vi "Main.vi"() -> ()   [LabVIEW 2017]
doc: "\"Discrete LED demo.vi\" -- Demonstrate a discrete LED connected to a digital output.\n\nInstructions:\n\n-- Click the 'enable blinker' button to toggle between blinking mode\nand static mode.\n-- In static mode, click the 'digital level' button to set the state of the\ndigital output.\n-- The 'digital output state' LED indicator shows the state of the\ndigital output (on = high, off = low)."
uses:
  <vilib>/myRIO/Instrument Drivers/Onboard IO/PWM/typedefs/PWM Reference.ctl
  <vilib>/myRIO/Common/Instrument Driver Framework/Utilities/typedefs/myRIO Generic Hardware Reference.ctl
  <vilib>/myRIO/Common/Instrument Driver Framework/Utilities/typedefs/Hardware Version Enum.ctl
  <vilib>/myRIO/Common/Instrument Driver Framework/Utilities/typedefs/myRIO v1.0 Reference.ctl
  <vilib>/myRIO/Common/Instrument Driver Framework/Utilities/typedefs/Generic FPGA Reference.ctl
  <vilib>/myRIO/Common/Instrument Driver Framework/myRIO v1.0/PWM/typedefs/PWM Channels Enum.ctl
  <vilib>/myRIO/Instrument Drivers/Onboard IO/PWM/typedefs/PWM Configuration.ctl
  <vilib>/userdefined/High Color/nirio_resource_hc.ctl
  <vilib>/myRIO/Instrument Drivers/Onboard IO/DIO/typedefs/DIO Reference.ctl
  <vilib>/myRIO/Common/Instrument Driver Framework/myRIO v1.0/DIO/typedefs/DIO Channels List.ctl
  <vilib>/myRIO/Common/Instrument Driver Framework/myRIO v1.0/DIO/typedefs/DIO Channels Enum.ctl
  <vilib>/myRIO/Common/Instrument Driver Framework/Utilities/vis/Is FPGA Ref Available.vi
  <vilib>/myRIO/Common/Instrument Driver Framework/myRIO v1.0/PWM/vis/myRIO v1.1 Open PWM.vi
  <vilib>/myRIO/Instrument Drivers/Onboard IO/PWM/vis/Set Duty Cycle and Frequency.vi
  <vilib>/myRIO/Common/Instrument Driver Framework/myRIO v1.0/DIO/vis/myRIO v1.1 Open DIO.vi
  <vilib>/myRIO/Instrument Drivers/Onboard IO/DIO/vis/Write.vi
  <vilib>/myRIO/Common/Instrument Driver Framework/Utilities/vis/Validate Channels.vi
  <vilib>/myRIO/Common/Instrument Driver Framework/myRIO v1.0/PWM/vis/myRIO v1.0 Reserve PWM.vi
  <vilib>/myRIO/Common/Instrument Driver Framework/myRIO v1.0/DIO/vis/myRIO v1.0 Reserve DIO.vi
  <vilib>/myRIO/Common/Instrument Driver Framework/myRIO v1.0/UART/vis/myRIO v1.0 Close UART.vi
  <vilib>/myRIO/Common/Instrument Driver Framework/myRIO v1.0/PWM/vis/myRIO v1.0 Build MUX Configuration PWM.vi
  <vilib>/myRIO/Common/Instrument Driver Framework/myRIO v1.0/Resource Manager/vis/myRIO v1.0 Reserve Channel List.vi
  <vilib>/myRIO/Common/Instrument Driver Framework/myRIO v1.0/DIO/vis/myRIO v1.0 Build MUX Configuration DIO.vi
  <vilib>/myRIO/Common/Instrument Driver Framework/myRIO v1.0/Resource Manager/vis/myRIO v1.0 Create Configuration List.vi
  <vilib>/myRIO/Common/Instrument Driver Framework/myRIO v1.0/Resource Manager/vis/myRIO v1.0 Reserve Channel.vi
  <vilib>/myRIO/Common/Instrument Driver Framework/myRIO v1.0/Resource Manager/vis/myRIO v1.0 Unreserve Channel.vi
  <vilib>/myRIO/Common/Instrument Driver Framework/myRIO v1.0/Resource Manager/vis/myRIO v1.0 Build Mutex Name.vi
  <vilib>/Utility/VariantDataType/GetNumericInfo.vi
  <vilib>/Utility/error.llb/Error Cluster From Error Code.vi
  <vilib>/myRIO/Common/Instrument Driver Framework/myRIO v1.0/myRIO v1.1 Open.vi
  <vilib>/myRIO/Common/Instrument Driver Framework/Utilities/vis/IO Manager.vi
  <vilib>/myRIO/Common/Instrument Driver Framework/Utilities/vis/Configuration Manager.vi
  <vilib>/myRIO/Common/Instrument Driver Framework/myRIO v1.0/Resource Manager/vis/myRIO v1.0 Configure IO.vi
  <vilib>/myRIO/Common/Instrument Driver Framework/myRIO v1.0/myRIO v1.0 Close.vi
  <vilib>/myRIO/Common/Instrument Driver Framework/myRIO v1.0/PWM/vis/myRIO v1.0 Write PWM.vi
  <vilib>/myRIO/Common/Instrument Driver Framework/myRIO v1.0/DIO/vis/myRIO v1.0 Write DIO.vi
  <vilib>/myRIO/Common/Instrument Driver Framework/Utilities/vis/FPGA Ref Manager.vi
  <vilib>/myRIO/Common/Instrument Driver Framework/myRIO v1.0/myRIO v1.0 Reset FPGA.vi
  <vilib>/myRIO/Common/Instrument Driver Framework/myRIO v1.0/IRQ/vis/myRIO v1.0 IRQ Info FGV.vi
  <vilib>/myRIO/Common/Instrument Driver Framework/myRIO v1.0/IRQ/vis/myRIO v1.0 Timer IRQ Info FGV.vi
  <vilib>/myRIO/Common/Instrument Driver Framework/myRIO v1.0/IRQ/vis/myRIO v1.0 ISR Agent.vi
  <vilib>/myRIO/Express VI/Onboard IO/PWM/PWM Express VI.xnode
  <vilib>/myRIO/Instrument Drivers/Onboard IO/PWM/vis/myRIO PWM Open.xnode
  <vilib>/myRIO/Express VI/Onboard Devices/LED/LED Express VI.xnode
  <vilib>/myRIO/Instrument Drivers/Onboard IO/DIO/vis/myRIO DIO Open.xnode
  <vilib>/myRIO/Express VI/Onboard IO/DO/DO Express VI.xnode
  <vilib>/myRIO/Instrument Drivers/Utilities/Utilities.lvlib
  <vilib>/myRIO/Instrument Drivers/Onboard IO/PWM/PWM.lvlib
  <vilib>/myRIO/Instrument Drivers/Onboard IO/DIO/DIO.lvlib
panel:
  in  "millisecond timer value":u32=100
  in  "PWM 2":dbl(slide)=0.5 scale=0.0..1.0
  in  "PWM 1":dbl(slide)=0.5 scale=0.0..1.0
  in  "Stop Button":bool
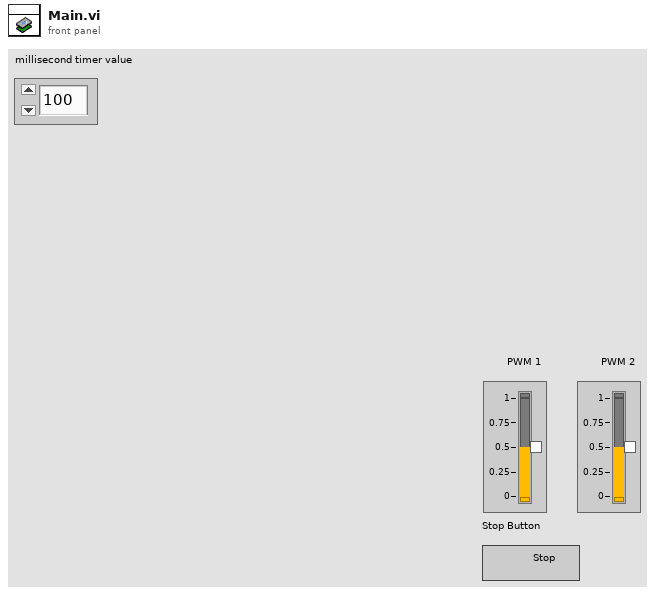
[diagram p1: front panel]
types:
  T1 = enum16{"0", "1", "2", "3", "4", "5", "6", "7", "8", "9", "A", "B", "C", "D", "E", "F", "G", "H", "I", "J", "K", "L", "M", "N", "O", "P", "Q", "R", "S", "T", "U", "V", "W", "X", "Y", "Z", "F1", "F2", "F3", "F4", "F5", "F6", "F7", "F8", "F9", "F10", "F11", "F12", "F13", "F14", "F15", "ADD", "BACK", "BACKSLASH", "CAPITAL", "COMMA", "DECIMAL", "DELETE", "DIVIDE", "DOWN", "END", "EQUALS", "ESCAPE", "GRAVE (`)", "HOME", "INSERT", "LBRACKET", "LCONTROL", "LEFT", "L ALT", "LSHIFT", "LWIN", "MINUS", "MULTIPLY", "NEXT", "NUMLOCK", "NUMPAD_0", "NUMPAD_1", "NUMPAD_2", "NUMPAD_3", "NUMPAD_4", "NUMPAD_5", "NUMPAD_6", "NUMPAD_7", "NUMPAD_8", "NUMPAD_9", "PAUSE", "PERIOD", "PRIOR (PG UP)", "RBRACKET", "RCONTROL", "RETURN", "RIGHT", "R ALT", "RSHIFT", "RWIN", "SCROLL", "SEMICOLON", "SLASH", "SPACE", "SUBTRACT", "TAB", "UP", "ENTER (num pad)", "' (quote)"}
  T2 = typedef "DIO.lvlib/DIO Reference.ctl" = cluster{"myRIO Reference":T3, "DIO Channels List":T7}
  T3 = typedef "myRIO Generic Hardware Reference.ctl" = cluster{"myRIO Model":T4, "myRIO Hardware Reference":T5}
  T4 = typedef "Hardware Version Enum.ctl" = enum16{"Unknown", "myRIO-1900", "myRIO-1950", "roboRIO", "NI ELVIS RIO CM"}
  T5 = typedef "myRIO v1.0 Reference.ctl" = cluster{"Generic FPGA Reference":T6, "Allow multiple opens":bool}
  T6 = typedef "Generic FPGA Reference.ctl" = refnum<k20>
  T7 = typedef "DIO Channels List.ctl" = T8[]
  T8 = typedef "DIO Channels Enum.ctl" = enum16{"Not Connected", "C/DIO0", "C/DIO1", "C/DIO2", "C/DIO3", "C/DIO4", "C/DIO5", "C/DIO6", "C/DIO7", "A/DIO0", "A/DIO1", "A/DIO2", "A/DIO3", "A/DIO4", "A/DIO5", "A/DIO6", "A/DIO7", "A/DIO8", "A/DIO9", "A/DIO10", "A/DIO11", "A/DIO12", "A/DIO13", "A/DIO14", "A/DIO15", "B/DIO0", "B/DIO1", "B/DIO2", "B/DIO3", "B/DIO4", "B/DIO5", "B/DIO6", "B/DIO7", "B/DIO8", "B/DIO9", "B/DIO10", "B/DIO11", "B/DIO12", "B/DIO13", "B/DIO14", "B/DIO15", "LED0", "LED1", "LED2", "LED3", "Button0", "DIO/DIO0", "DIO/DIO1", "DIO/DIO2", "DIO/DIO3", "DIO/DIO4", "DIO/DIO5", "DIO/DIO6", "DIO/DIO7", "DIO/DIO8", "DIO/DIO9", "SPI/CS0", "SPI/CS1", "SPI/CS2", "SPI/CS3", "LED RADIO (Green)", "LED RADIO (Red)", "LED COMM (Green)", "LED COMM (Red)", "LED MODE (Green)", "LED MODE (Red)"}
  T9 = typedef "nirio_resource_hc.ctl" = tag
  T10 = typedef "PWM.lvlib/PWM Reference.ctl" = cluster{"myRIO Reference":T3, "PWM Channels Enum":T11, "PWM Configuration":T12}
  T11 = typedef "PWM Channels Enum.ctl" = enum16{"Not Connected", "C/PWM0", "C/PWM1", "A/PWM0", "A/PWM1", "A/PWM2", "B/PWM0", "B/PWM1", "B/PWM2", "PWM/PWM0", "PWM/PWM1", "PWM/PWM2", "PWM/PWM3", "PWM/PWM4", "PWM/PWM5", "PWM/PWM6", "PWM/PWM7", "PWM/PWM8", "PWM/PWM9"}
  T12 = typedef "PWM.lvlib/PWM Configuration.ctl" = cluster{"Frequency":dbl, "Duty Cycle":dbl}
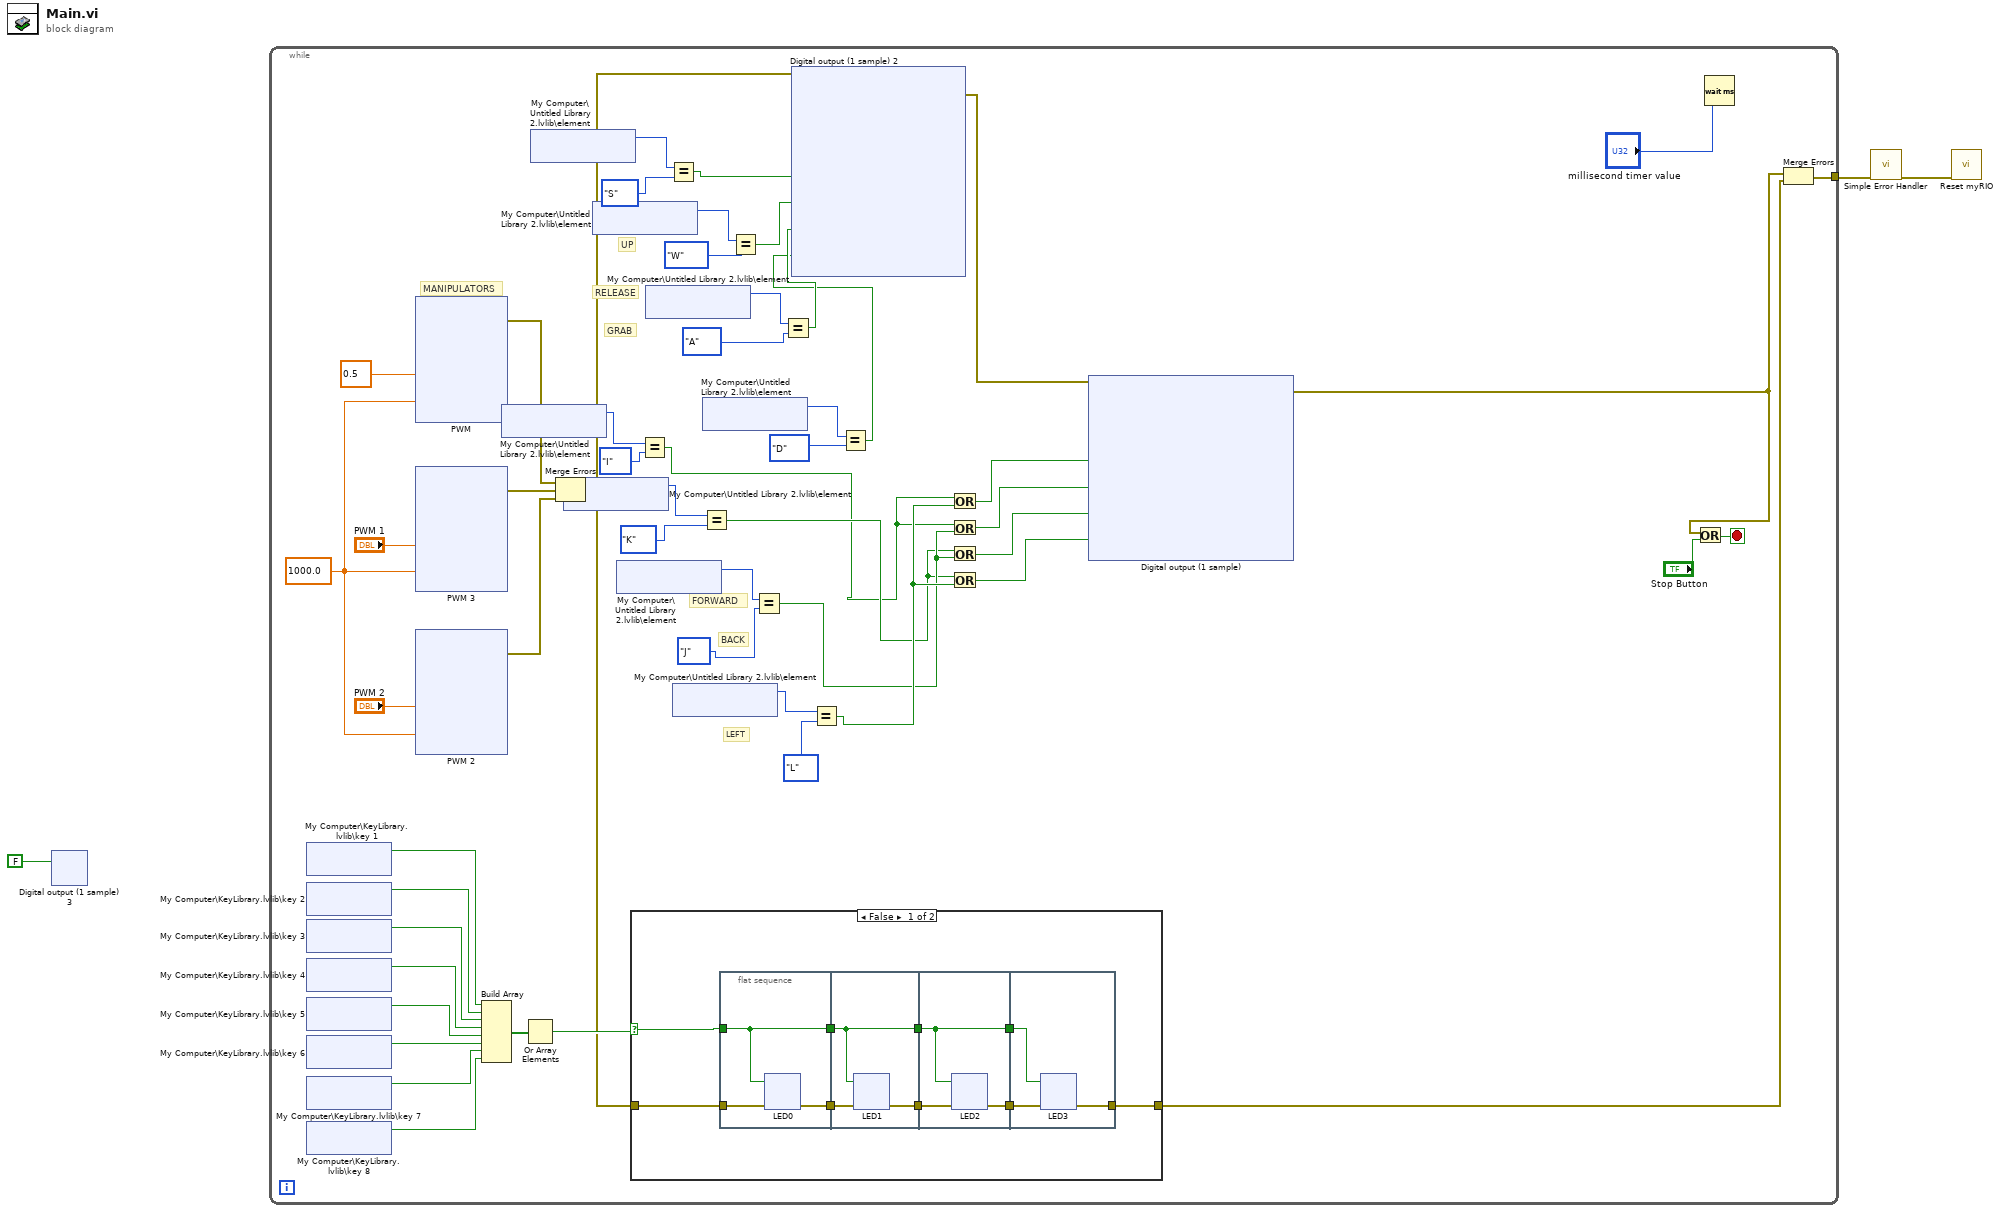
[diagram p0: block diagram]
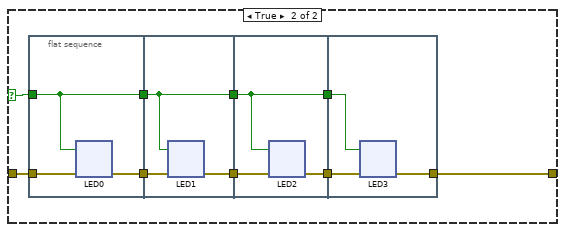
[diagram p2: hidden frame]
diagram:
  n1 = xnode "Digital output (1 sample) 3"("LED_pos (A/DIO2 (Pin 15))"=FALSE) -> ()  [unwired: 1 in, 1 out]
  n2 = while {
    tunnel: [w35] -> w2
    stop <- w55 stop-if-true
    w29 = 1000.0 ("Frequency [Hz]")
    # "RELEASE"
    # "GRAB"
    # "DOWN"
    # "UP"
    # "LEFT"
    # "RIGHT"
    # "BACK"
    # "FORWARD"
    # "MANIPULATORS"
    n3 = shared-variable "My Computer\\KeyLibrary.lvlib\\key 1"() -> (w45:bool)  [unwired: 1 in, 1 out]
    n4 = shared-variable "My Computer\\KeyLibrary.lvlib\\key 2"() -> (w44:bool)  [unwired: 1 in, 1 out]
    n5 = shared-variable "My Computer\\KeyLibrary.lvlib\\key 3"() -> (w43:bool)  [unwired: 1 in, 1 out]
    n6 = shared-variable "My Computer\\KeyLibrary.lvlib\\key 4"() -> (w42:bool)  [unwired: 1 in, 1 out]
    n7 = shared-variable "My Computer\\KeyLibrary.lvlib\\key 5"() -> (w41:bool)  [unwired: 1 in, 1 out]
    n8 = shared-variable "My Computer\\KeyLibrary.lvlib\\key 6"() -> (w40:bool)  [unwired: 1 in, 1 out]
    n9 = shared-variable "My Computer\\KeyLibrary.lvlib\\key 7"() -> (w39:bool)  [unwired: 1 in, 1 out]
    n10 = shared-variable "My Computer\\KeyLibrary.lvlib\\key 8"() -> (w38:bool)  [unwired: 1 in, 1 out]
    n11 = xnode "PWM"("Duty Cycle"=0.5, "Frequency [Hz]"=w29) -> ("error out"=w51:errorcluster)  [unwired: 1 in]
    n12 = xnode "PWM 3"("Duty Cycle"="PWM 1", "Frequency [Hz]"=w29) -> ("error out"=w54:errorcluster)  [unwired: 1 in]
    n13 = xnode "PWM 2"("Duty Cycle"="PWM 2", "Frequency [Hz]"=w29) -> ("error out"=w53:errorcluster)  [unwired: 1 in]
    n14 = Build Array(w45, w44, w43, w42, w41, w40, w39, w38) -> (w37:bool[])
    n15 = shared-variable "My Computer\\Untitled Library 2.lvlib\\element"() -> (w19:T1)  [unwired: 1 in, 1 out]
    n16 = Or Array Elements(Boolean array=w37) -> (logical OR=w36:bool)
    n17 = shared-variable "My Computer\\Untitled Library 2.lvlib\\element"() -> (w27:T1)  [unwired: 1 in, 1 out]
    n18 = Merge Errors(w51, w54, w53) -> (w33:errorcluster)
    n19 = shared-variable "My Computer\\Untitled Library 2.lvlib\\element"() -> (w18:T1)  [unwired: 1 in, 1 out]
    n20 = shared-variable "My Computer\\Untitled Library 2.lvlib\\element"() -> (w25:T1)  [unwired: 1 in, 1 out]
    n21 = shared-variable "My Computer\\Untitled Library 2.lvlib\\element"() -> (w17:T1)  [unwired: 1 in, 1 out]
    n22 = case shown="False" w36 {
      selector: w36 -> [w57 w226]
      tunnel: [w58 w218] -> w34
      tunnel: w33 -> [w59 w219]
      frame False {
        n23 = flat-sequence {
          tunnel: w57 -> [w66]
          tunnel: [w66] -> w65
          tunnel: [w68] -> w64
          tunnel: w59 -> [w67]
          tunnel: [w106] -> w63
          tunnel: w65 -> [w106]
          tunnel: w64 -> [w105]
          tunnel: [w104] -> w62
          tunnel: [w144] -> w61
          tunnel: w63 -> [w144]
          tunnel: w62 -> [w143]
          tunnel: [w142] -> w60
          tunnel: w61 -> [w182]
          tunnel: w60 -> [w181]
          tunnel: [w180] -> w58
          frame #0 {
            n24 = xnode "LED0"("error in (no error)"=w67, "LED0"=w66) -> ("error out"=w68:errorcluster)
          }
          frame #1 {
            n25 = xnode "LED1"("error in (no error)"=w105, "LED1"=w106) -> ("error out"=w104:errorcluster)
          }
          frame #2 {
            n26 = xnode "LED2"("error in (no error)"=w143, "LED2"=w144) -> ("error out"=w142:errorcluster)
          }
          frame #3 {
            n27 = xnode "LED3"("error in (no error)"=w181, "LED3"=w182) -> ("error out"=w180:errorcluster)
          }
        }
      }
      frame True {
        n28 = flat-sequence {
          tunnel: w226 -> [w229]
          tunnel: [w229] -> w223
          tunnel: [w228] -> w222
          tunnel: w219 -> [w227]
          tunnel: [w267] -> w224
          tunnel: w223 -> [w267]
          tunnel: w222 -> [w266]
          tunnel: [w265] -> w221
          tunnel: [w305] -> w225
          tunnel: w224 -> [w305]
          tunnel: w221 -> [w304]
          tunnel: [w303] -> w220
          tunnel: w225 -> [w343]
          tunnel: w220 -> [w342]
          tunnel: [w341] -> w218
          frame #0 {
            n29 = xnode "LED0"("error in (no error)"=w227, "LED0"=w229) -> ("error out"=w228:errorcluster)
          }
          frame #1 {
            n30 = xnode "LED1"("error in (no error)"=w266, "LED1"=w267) -> ("error out"=w265:errorcluster)
          }
          frame #2 {
            n31 = xnode "LED2"("error in (no error)"=w304, "LED2"=w305) -> ("error out"=w303:errorcluster)
          }
          frame #3 {
            n32 = xnode "LED3"("error in (no error)"=w342, "LED3"=w343) -> ("error out"=w341:errorcluster)
          }
        }
      }
    }
    n33 = Equal?(x=w19, y=T1."I") -> (x = y?=w12:bool)
    n34 = shared-variable "My Computer\\Untitled Library 2.lvlib\\element"() -> (w23:T1)  [unwired: 1 in, 1 out]
    n35 = Equal?(x=w27, y=T1."S") -> (x = y?=w26:bool)
    n36 = shared-variable "My Computer\\Untitled Library 2.lvlib\\element"() -> (w16:T1)  [unwired: 1 in, 1 out]
    n37 = Equal?(x=w18, y=T1."K") -> (x = y?=w13:bool)
    n38 = shared-variable "My Computer\\Untitled Library 2.lvlib\\element"() -> (w21:T1)  [unwired: 1 in, 1 out]
    n39 = Equal?(x=w25, y=T1."W") -> (x = y?=w24:bool)
    n40 = Equal?(x=w17, y=T1."J") -> (x = y?=w14:bool)
    n41 = Equal?(x=w23, y=T1."A") -> (x = y?=w22:bool)
    n42 = Equal?(x=w16, y=T1."L") -> (x = y?=w15:bool)
    n43 = Equal?(x=w21, y=T1."D") -> (x = y?=w20:bool)
    n44 = xnode "Digital output (1 sample) 2"("M+ (B/DIO5 (Pin 21))"=w26, "M- (B/DIO6 (Pin 23))"=w24, "G+ (B/DIO7 (Pin 25))"=w22, "G- (B/DIO13 (Pin 26))"=w20, "error in (no error)"=w33) -> ("error out"=w49:errorcluster)
    n45 = Or(x=w12, y=w15) -> (x .or. y?=w47:bool)
    n46 = Or(x=w12, y=w14) -> (x .or. y?=w30:bool)
    n47 = Or(x=w13, y=w14) -> (x .or. y?=w31:bool)
    n48 = Or(x=w13, y=w15) -> (x .or. y?=w46:bool)
    n49 = xnode "Digital output (1 sample)"("Left+ (A/DIO5 (Pin 21))"=w47, "Right+ (A/DIO7 (Pin 25))"=w30, "Left- (A/DIO6 (Pin 23))"=w31, "Right- (A/DIO13 (Pin 26))"=w46, "error in (no error)"=w49) -> ("error out"=w32:errorcluster)
    n50 = Or(x=w32, y="Stop Button") -> (x .or. y?=w55:bool)
    n51 = Wait (ms)(milliseconds to wait="millisecond timer value") -> ()  [unwired: 1 out]
    n52 = Merge Errors(w32, w34) -> (w35:errorcluster)
  }
  n53 = call <vilib>:"Simple Error Handler.vi"("error in (no error)"=w2) -> ("error out"=w3:errorcluster)  [unwired: 4 in, 4 out]
  n54 = call <vilib>:"Reset myRIO.vi"("error in (no error)"=w3) -> ()  [unwired: 10 in, 1 out]
